vi "Get Local UTC Offset.vi"(9 "timestamp (now)":timestamp, 10 "UTC? (F)":bool) -> (1 "UTC Offset String":string, 2 "UTC Offset":T1=enum."UTC+00:00")   [LabVIEW 2013]
uses:
  UTC Offsets -- enum.ctl
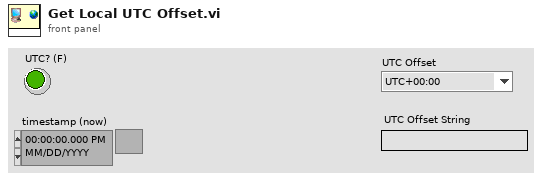
[diagram p1: front panel]
types:
  T1 = typedef "UTC Offsets -- enum.ctl" = enum16{"UTC-12:00", "UTC-11:00", "UTC-10:00", "UTC-09:30", "UTC-09:00", "UTC-08:00", "UTC-07:00", "UTC-06:00", "UTC-05:00", "UTC-04:00", "UTC-03:30", "UTC-03:00", "UTC-02:00", "UTC-01:00", "UTC-00:00", "UTC+00:00", "UTC+01:00", "UTC+02:00", "UTC+03:00", "UTC+03:30", "UTC+04:00", "UTC+04:30", "UTC+05:00", "UTC+05:30", "UTC+05:45", "UTC+06:00", "UTC+06:30", "UTC+07:00", "UTC+08:00", "UTC+08:45", "UTC+09:00", "UTC+09:30", "UTC+10:00", "UTC+10:30", "UTC+11:00", "UTC+12:00", "UTC+12:45", "UTC+13:00", "UTC+14:00"}
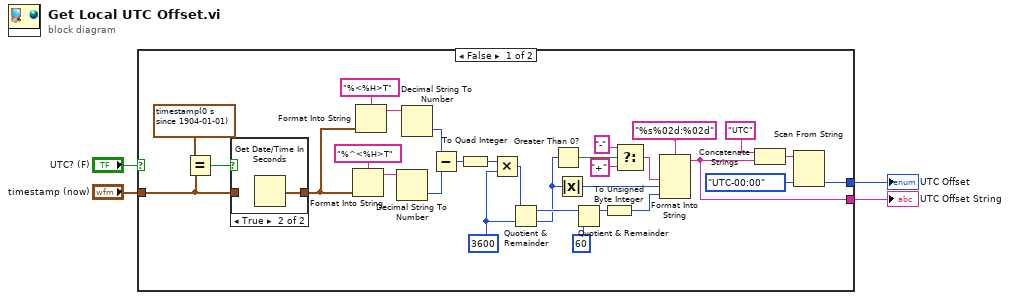
[diagram p0: block diagram]
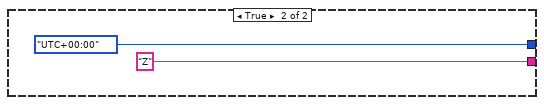
[diagram p3: hidden frame]
diagram:
  n1 = case shown="False" "UTC? (F)" {
    tunnel: [w34 UTC_Offsets_--_enum."UTC+00:00" ("UTC Time Offset")] -> w4
    tunnel: [w33 "Z"] -> w3
    tunnel: "timestamp (now)" -> [w6 _]
    frame False {
      w11 = i64 3600 ("y")
      n2 = Equal?(x=timestamp(0 s since 1904-01-01), y=w6) -> (x = y?=w8:bool)
      n3 = case shown="True" w8 {
        tunnel: [w35 w36] -> w5
        tunnel: w6 -> [w35 _]
        frame False {
        }
        frame True {
          n4 = Get Date/Time In Seconds() -> (seconds since 1Jan1904=w36:timestamp)
        }
      }
      n5 = Format Into String(format string="%^<%H>T", w5) -> (resulting string=w15:string)  [unwired: 2 in, 1 out]
      n6 = Format Into String(format string="%<%H>T", w5) -> (resulting string=w16:string)  [unwired: 2 in, 1 out]
      n7 = Decimal String To Number(string=w15) -> (number=w13:i32)  [unwired: 2 in, 1 out]
      n8 = Decimal String To Number(string=w16) -> (number=w14:i32)  [unwired: 2 in, 1 out]
      n9 = Subtract(x=w14, y=w13) -> (x-y=w12:i32)
      n10 = To Quad Integer(1:w12) -> (0:w9:i64)
      n11 = Multiply(x=w9, y=w11) -> (x*y=w10:i64)
      n12 = Quotient & Remainder(x=w10, y=w11) -> (x-y*floor(x/y)=w25:i64, floor(x/y)=w23:i64)
      n13 = Greater Than 0?(x=w23) -> (x > 0?=w29:bool)
      n14 = Absolute Value(x=w23) -> (abs(x)=w26:i64)
      n15 = Quotient & Remainder(x=w25, y=i64 60) -> (x-y*floor(x/y)=w32:i64)  [unwired: 1 out]
      n16 = To Unsigned Byte Integer(number=w32) -> (unsigned 8bit integer=w31:u8)
      n17 = Select(t="-" ("format string"), s=w29, f="+" ("format string")) -> (s? t:f=w21:string)
      n18 = Format Into String(format string="%s%02d:%02d", w21, w26, w31) -> (resulting string=w33:string)  [unwired: 2 in, 1 out]
      n19 = Concatenate Strings("UTC" ("format string"), w33) -> (w20:string)
      n20 = Scan From String(input string=w20, default 1=UTC_Offsets_--_enum."UTC-00:00" ("UTC Time Offset")) -> (output 1=w34:T1)  [unwired: 3 in, 3 out]
    }
    frame True {
    }
  }
  "UTC Offset" <- w4
  "UTC Offset String" <- w3
